vi "Change Desired Temperature.vi"(8 "error in (no error)":errorcluster, 10 "Desired Temperature":dbl=75.0, 11 "Cooler UI with Events in":refnum<class "Cooler UI with Events.lvclass">=refnum) -> (0 "error out":errorcluster, 3 "Cooler UI with Events out":refnum<class "Cooler UI with Events.lvclass">)   [LabVIEW 2012, in "Cooler UI.lvlib" / "Cooler UI with Events.lvclass"]
uses:
  Cooler UI with Events.lvclass
  Cooler UI with Events.lvclass/Cooler UI with Events.ctl
  Level Controller/Write Deadband Msg/Write Deadband Msg.lvclass/Write Deadband Msg.ctl
  <vilib>/ActorFramework/Message Enqueuer/Message Enqueuer.lvclass/Message Enqueuer.ctl
  <vilib>/ActorFramework/Message Enqueuer/Enqueue.vi
  <vilib>/ActorFramework/Message Priority Queue/Priority Enqueue.vi
  Level Controller/Write Deadband Msg/Write Deadband Msg.lvclass
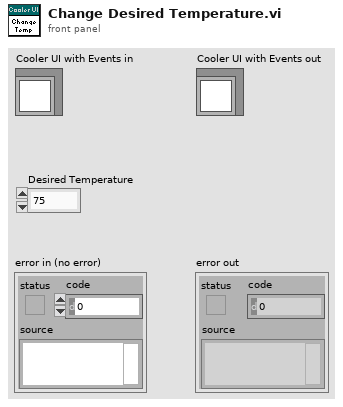
[diagram p1: front panel]
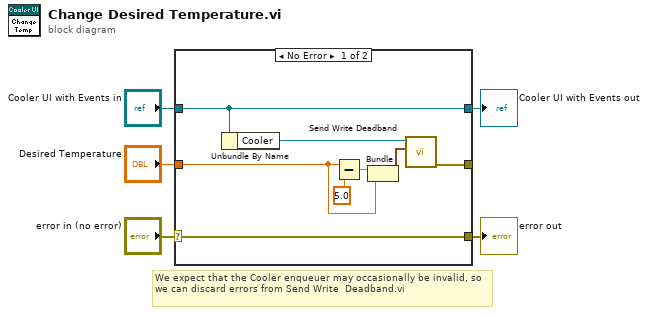
[diagram p0: block diagram]
diagram:
  # "We expect that the Cooler enqueuer may occasionally be invalid, so we can discard errors from Send Write  Deadband.vi"
  n1 = case shown="No Error" "error in (no error)" {
    selector: "error in (no error)" -> [w13 w15]
    tunnel: [w13 w15] -> w4
    tunnel: [w12 w14] -> w2
    tunnel: "Cooler UI with Events in" -> [w12 w14]
    tunnel: "Desired Temperature" -> [w7 _]
    tunnel: [w6 _] -> _
    frame No Error {
      n2 = Unbundle By Name(w12) -> ("Cooler"=w8:refnum<class "Message Enqueuer.lvclass">)
      n3 = Subtract(x=w7, y=5.0) -> (x-y=w10:dbl)
      n4 = Bundle(w10, "Desired Temperature"=w7) -> (w11:cluster{dbl, "Desired Temperature":dbl})  [unwired: 1 in]
      n5 = call "Send Write Deadband.vi"("Deadband"=w11, "enqueuer"=w8) -> ("error out"=w6:errorcluster)  [unwired: 9 in]
    }
    frame Error {
    }
  }
  "error out" <- w4
  "Cooler UI with Events out" <- w2
